vi "Init Modal Window.vi"(4 "Window Vertical Size (pixels)":i16=600, 6 "Window Horizontal Size (pixels)":i16=800, 7 "Window Close (X) Button Enabled? (Default = True)":bool=TRUE, 8 "Error In":errorcluster, 9 "Background Colour (Default = 255,255,255)":u32(colorbox)=16777215, 10 "Window Title":string="Modal Dialogue", 11 "VI Refnum":refnum<vi>) -> (0 "Error Out":errorcluster)   [LabVIEW 2023, in "Error Manager.lvlib"]
doc: "This VI configures the Front Panel (the GUI Window) of the VI whose refnum is passed as an argument to the \"VI Refnum\" input (usually, the immediate caller VI)."
uses:
  Error Manager.lvlib
  <vilib>/Utility/miscctls.llb/LVPointTypeDef.ctl
  <vilib>/Utility/miscctls.llb/LVRectTypeDef.ctl
panel:
  # "Development\ncontrols/indicators useful for development and testing, but which are not outputs of the VI"
  # "Input\nInputs to the VI"
  # "Output\nOutputs of the VI"
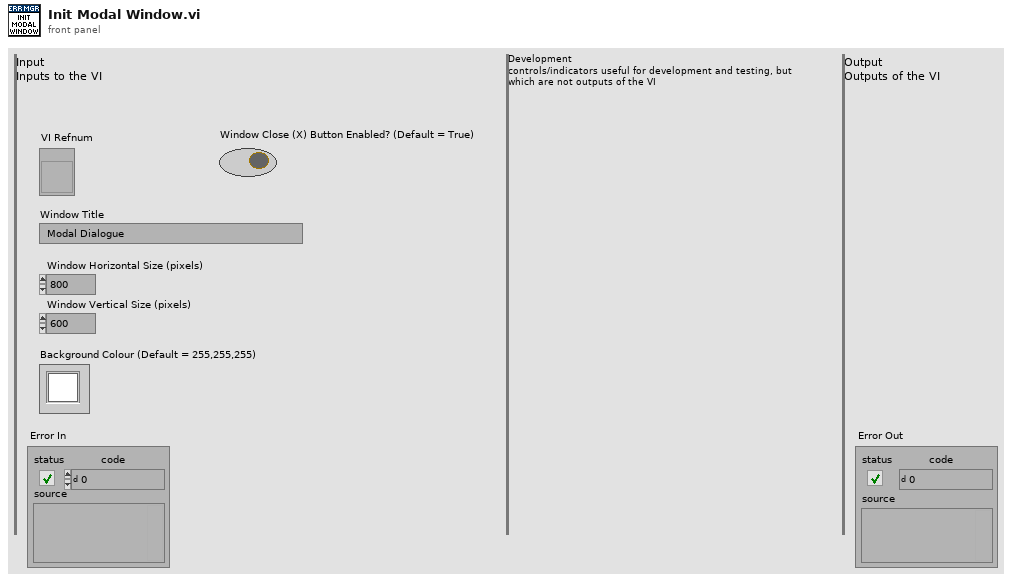
[diagram p1: front panel]
types:
  T1 = enum32{"Invalid", "Standard", "Closed", "Hidden", "Minimized", "Maximized"}
  T2 = typedef "LVRectTypeDef.ctl" = cluster{"Left":i16, "Top":i16, "Right":i16, "Bottom":i16}
  T3 = typedef "LVPointTypeDef.ctl" = cluster{"Horizontal":i16, "Vertical":i16}
  T4 = enum32{"Invalid", "Default", "Floating", "Floating/Auto-Hide", "Modal"}
  T5 = enum16{"Always On", "Always Off", "Off While Running"}
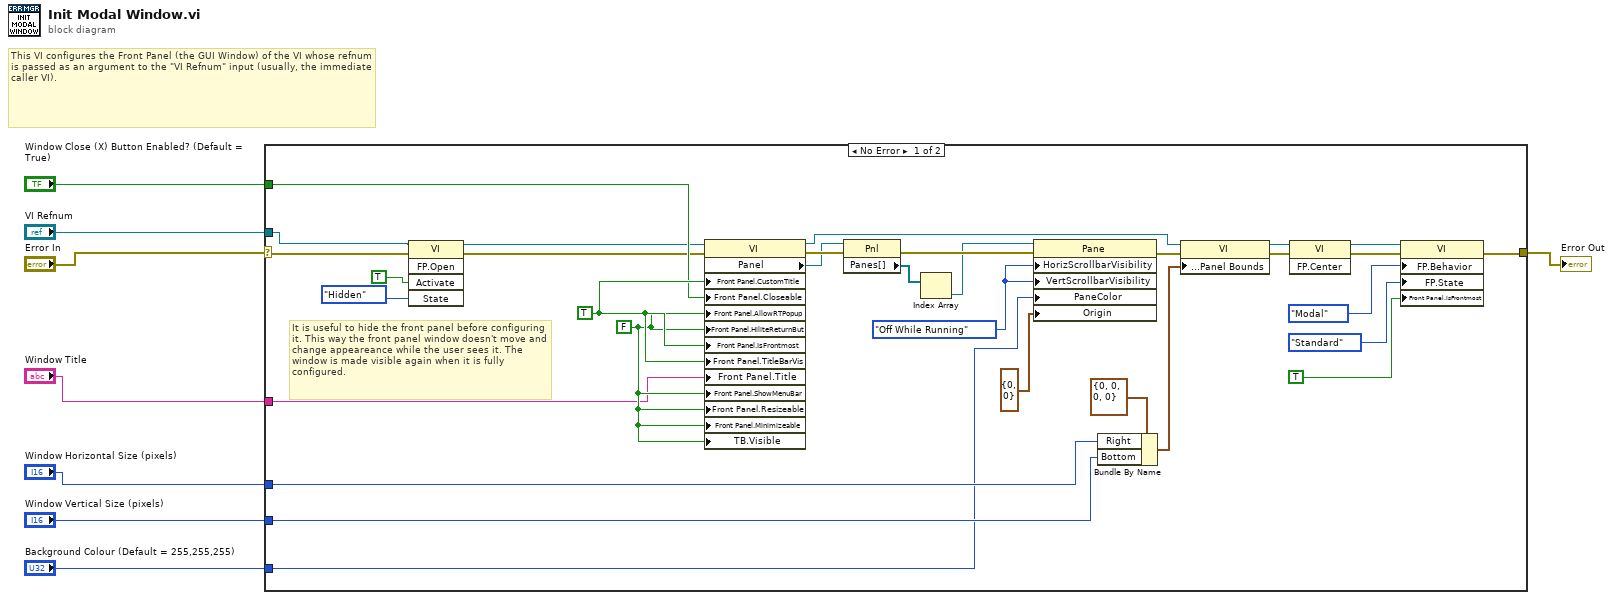
[diagram p0: block diagram]
diagram:
  # "This VI configures the Front Panel (the GUI Window) of the VI whose refnum is passed as an argument to the \"VI Refnum\" input (usually, the immediate caller VI)."
  n1 = case shown="No Error" "Error In" {
    selector: "Error In" -> [w18 w41]
    tunnel: [w12 w41] -> w7
    tunnel: "VI Refnum" -> [w16 _]
    tunnel: "Window Title" -> [w25 _]
    tunnel: "Window Horizontal Size (pixels)" -> [w24 _]
    tunnel: "Window Vertical Size (pixels)" -> [w23 _]
    tunnel: "Window Close (X) Button Enabled? (Default = True)" -> [w22 _]
    tunnel: "Background Colour (Default = 255,255,255)" -> [w21 _]
    frame No Error {
      w34 = T5."Off While Running" ("Horizontal Scrollbar Visibility")
      w33 = FALSE
      w39 = TRUE
      # "It is useful to hide the front panel before configuring it. This way the front panel window doesn't move and change appeareance while the user sees it. The window is made visible again when it is fully configured."
      n2 = invoke class="VI" method="FP.Open"(reference=w16, error in=w18, "Activate"=TRUE ("Activate?"), "State"=T1."Hidden") -> (reference out=w15:refnum<vi>, error out=w17:errorcluster)  [unwired: 1 in, 3 out]
      n3 = property class="VI"(reference=w15, error in=w17, "Front Panel.CustomTitle"=w39, "Front Panel.Closeable"=w22, "Front Panel.AllowRTPopup"=w33, "Front Panel.HiliteReturnBut"=w33, "Front Panel.IsFrontmost"=w39, "Front Panel.TitleBarVis"=w39, "Front Panel.Title"=w25, "Front Panel.ShowMenuBar"=w33, "Front Panel.Resizeable"=w33, "Front Panel.Minimizeable"=w33, "TB.Visible"=w33) -> (reference out=w29:refnum<vi>, error out=w40:errorcluster, "Panel"=w37:refnum<vi>)
      n4 = property class="Pnl"(reference=w37, error in=w40) -> (error out=w38:errorcluster, "Panes[]"=w36:refnum<vi>[])  [unwired: 1 out]
      n5 = Index Array(array=w36) -> (element=w35:refnum<vi>)  [unwired: 1 in]
      n6 = property class="Pane"(reference=w35, error in=w38, "HorizScrollbarVisibility"=w34, "VertScrollbarVisibility"=w34, "PaneColor"=w21, "Origin"=T3 {"Horizontal"=0, "Vertical"=0}) -> (error out=w31:errorcluster)  [unwired: 1 out]
      n7 = Bundle By Name(cluster=T2 {"Left"=0, "Top"=0, "Right"=0, "Bottom"=0} ("Front Panel Window:Panel Bounds"), "Right"=w24, "Bottom"=w23) -> (w27:T2)
      n8 = property on="Property Node" class="VI"(reference=w29, error in=w31, "Front Panel Window:Panel Bounds"=w27) -> (reference out=w26:refnum<vi>, error out=w30:errorcluster)
      n9 = invoke class="VI" method="FP.Center"(reference=w26, error in=w30) -> (reference out=w10:refnum<vi>, error out=w11:errorcluster)  [unwired: 1 in, 1 out]
      n10 = property class="VI"(reference=w10, error in=w11, "FP.Behavior"=T4."Modal" ("Front Panel Window:Behavior"), "FP.State"=T1."Standard" ("Front Panel Window:State"), "Front Panel.IsFrontmost"=TRUE ("Front Panel Window:Is Frontmost")) -> (error out=w12:errorcluster)  [unwired: 1 out]
    }
    frame Error {
    }
  }
  "Error Out" <- w7
